vi "ATF-Storage-Drive_Element to Waveform_A.vi"(11 "Array input":i16[](array[numeric])) -> (2 "RPM out":waveform(dbl)[](array[waveform]))   [LabVIEW 2022 SP3]
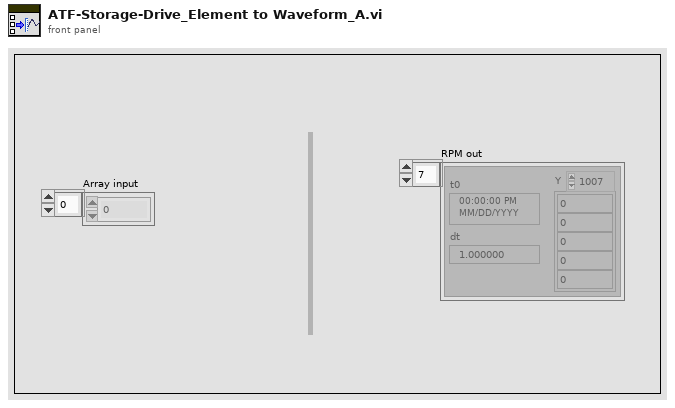
[diagram p1: front panel]
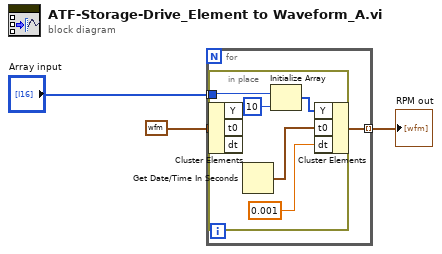
[diagram p0: block diagram]
diagram:
  n1 = for {
    tunnel: [w5] -> w2 mode=indexing
    tunnel: waveform(dbl) {"t0"=timestamp(0 s since 1904-01-01), "dt"=0.001, "Y"=[]} ("Waveform") -> [w6]
    tunnel: "Array input" -> [w4] mode=indexing
    n2 = in-place {
      in-place-border: w4 -> [w9]
      n3 = in-place-cluster #1(w6) -> ()  [unwired: 3 out]
      n4 = Get Date/Time In Seconds() -> (seconds since 1Jan1904=w11:timestamp)
      n5 = Initialize Array(w9, 10 ("dimension size")) -> (w7:i16[])
      n6 = in-place-cluster #1("Y"=w7, "t0"=w11, "dt"=0.001) -> (w5:waveform(dbl))
    }
  }
  "RPM out" <- w2
